vi "Copy Acquisition.vi"(4 "error in (no error)":errorcluster, 7 "pDataBuffer":u16[](array[numeric])) -> (0 "error out":errorcluster, 2 "function return":i32, 3 "pDataBuffer":u16[](array[numeric]))   [LabVIEW 2020, in "ThorConfocal.lvlib"]
doc: "long CopyAcquisition(char * pDataBuffer);"
uses:
  ThorConfocal.lvlib
  ThorConfocal.dll
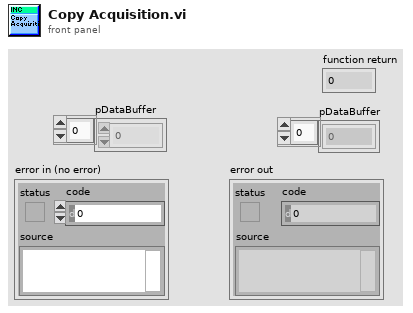
[diagram p1: front panel]
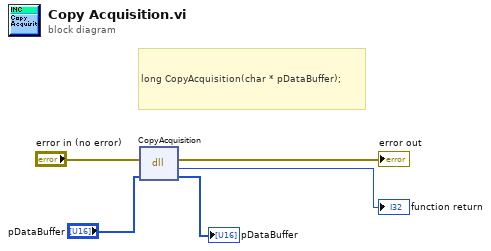
[diagram p0: block diagram]
diagram:
  # "long CopyAcquisition(char * pDataBuffer);"
  n1 = dll-call lib="D:/software/TweezerTron Project/Instruments/Thorlabs/LSM_SDK/ThorConfocal.dll" fn="CopyAcquisition"(error in="error in (no error)", "pDataBuffer"="pDataBuffer") -> (error out=→"error out":errorcluster, "return type"=→"function return":i32, "pDataBuffer"=→"pDataBuffer":u16[])  [unwired: 2 in, 1 out]
